vi "SelectProductsSabritas.vi"(8 "error in (no error)":errorcluster, 10 "Productos":i32(listbox), 11 "Sabritas Actor in":refnum<class "Sabritas Actor.lvclass">) -> (0 "error out":errorcluster, 3 "Sabritas Actor out":refnum<class "Sabritas Actor.lvclass">)   [LabVIEW 2020, in "Sabritas Actor.lvlib" / "Sabritas Actor.lvclass"]
uses:
  Sabritas Actor.lvclass
  C:/Program Files (x86)/National Instruments/LabVIEW 2020/vi.lib/ActorFramework/Actor/Actor.lvclass
  <vilib>/ActorFramework/Actor/Actor.lvclass/Actor.ctl
  Sabritas Actor.lvclass/Sabritas Actor.ctl
  UI Actor Messages/SelectProduct Msg/SelectProduct Msg.lvclass/SelectProduct Msg.ctl
  <vilib>/ActorFramework/Message Enqueuer/Message Enqueuer.lvclass/Message Enqueuer.ctl
  <vilib>/ActorFramework/Message Enqueuer/Enqueue.vi
  UI Actor Messages/SelectProduct Msg/SelectProduct Msg.lvclass
  C:/Program Files (x86)/National Instruments/LabVIEW 2020/vi.lib/ActorFramework/Message/Message.lvclass
  <vilib>/ActorFramework/Message Priority Queue/Priority Enqueue.vi
  <vilib>/ActorFramework/Actor/Actor.lvclass
panel:
  in  "Data":string[](array[string])
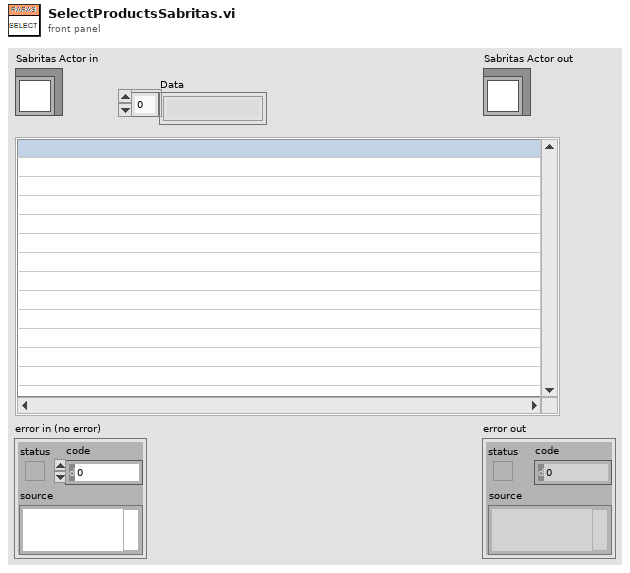
[diagram p1: front panel]
types:
  T1 = cluster{"Data[0]":string, "Data[1]":string, "Data[2]":string, "Data[3]":string, "Data[4]":string, "Data[5]":string, "Data[6]":string, "Data[7]":string, "Data[8]":string}
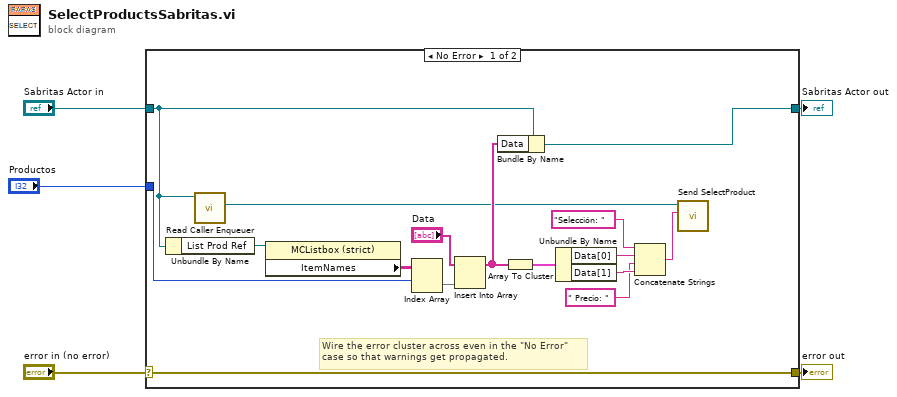
[diagram p0: block diagram]
diagram:
  n1 = case shown="No Error" "error in (no error)" {
    selector: "error in (no error)" -> [w21 w23]
    tunnel: [w21 w23] -> w4
    tunnel: [w8 w22] -> w2
    tunnel: "Sabritas Actor in" -> [w6 w22]
    tunnel: "Productos" -> [w7 _]
    frame No Error {
      # "Wire the error cluster across even in the \"No Error\"\ncase so that warnings get propagated."
      n2 = Unbundle By Name(w6) -> ("List Prod Ref"=w20:refnum<vi>)
      n3 = call <vilib>:"Read Caller Enqueuer.vi"("Actor"=w6) -> ("Caller Enqueuer"=w9:refnum<class "Message Enqueuer.lvclass">)  [unwired: 10 in]
      n4 = property class="MCListbox (strict)"(reference=w20) -> ("ItemNames"=w19:string[][])  [unwired: 1 in, 2 out]
      n5 = Index Array(array=w19, index (row)=w7) -> (element=w18:string[])  [unwired: 1 in]
      n6 = Insert Into Array(array="Data", new element=w18) -> (w16:string[])  [unwired: 1 in]
      n7 = Bundle By Name(cluster=w6, "Data"=w16) -> (w8:refnum<class "Sabritas Actor.lvclass">)
      n8 = Array To Cluster(array=w16) -> (cluster=w15:T1)
      n9 = Unbundle By Name(w15) -> ("Data[0]"=w14:string, "Data[1]"=w13:string)
      n10 = Concatenate Strings("Selección: " ("string"), w14, " Precio: " ("string"), w13) -> (w10:string)
      n11 = call "Send SelectProduct.vi"("Producto"=w10, "Message Enqueuer"=w9) -> ()  [unwired: 8 in, 2 out]
    }
    frame Error {
    }
  }
  "error out" <- w4
  "Sabritas Actor out" <- w2
